vi "Unescape HTTP URL.vi"(1 "escaped string in":string) -> (0 "unescaped string out":string)   [LabVIEW 2020, in "HTTP Utils.lvlib"]
uses:
  HTTP Utils.lvlib
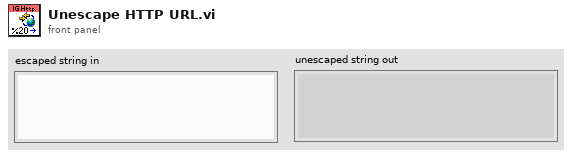
[diagram p1: front panel]
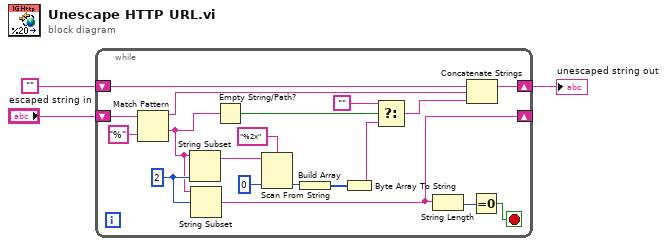
[diagram p0: block diagram]
diagram:
  n1 = while {
    shift-right: [w17] -> _
    shift-left: "escaped string in" -> [w22]
    shift-right: [w19] -> w1
    shift-left: "" -> [w18]
    stop <- w15 stop-if-true
    w20 = 2 ("length (rest)")
    n2 = Match Pattern(string=w22, regular expression="%") -> (before substring=w14:string, after substring=w5:string)  [unwired: 1 in, 2 out]
    n3 = String Subset(string=w5, length (rest)=w20) -> (substring=w11:string)  [unwired: 1 in]
    n4 = String Subset(string=w5, offset (0)=w20) -> (substring=w17:string)  [unwired: 1 in]
    n5 = Empty String/Path?(string/path=w5) -> (empty?=w9:bool)
    n6 = Scan From String(format string="%2x", input string=w11, default 1=u8 0) -> (output 1=w12:u8)  [unwired: 2 in, 3 out]
    n7 = Build Array(w12) -> (w10:u8[])
    n8 = Byte Array To String(unsigned byte array=w10) -> (string=w7:string)
    n9 = Select(t="", s=w9, f=w7) -> (s? t:f=w6:string)
    n10 = String Length(string=w17) -> (length=w16:i32)
    n11 = Concatenate Strings(w18, w14, w6) -> (w19:string)
    n12 = Equal To 0?(x=w16) -> (x = 0?=w15:bool)
  }
  "unescaped string out" <- w1
